vi "EnqueueError.vi"(8 "ErrorArray":errorcluster[](array[cluster])) -> (0 "ErrorArray":errorcluster[](array[cluster]))   [LabVIEW 2014, in "Bus_class.lvlib" / "Bus.lvclass"]
uses:
  Bus.lvclass
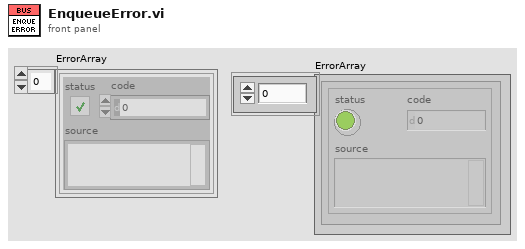
[diagram p1: front panel]
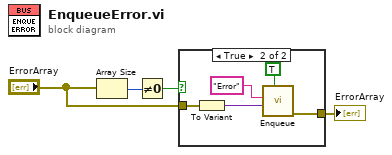
[diagram p0: block diagram]
diagram:
  n1 = Array Size(array="ErrorArray") -> (size(s)=w4:i32)
  n2 = Not Equal To 0?(x=w4) -> (x != 0?=w3:bool)
  n3 = case shown="True" w3 {
    tunnel: "ErrorArray" -> [_ w8]
    tunnel: [_ w5] -> w1
    frame False {
    }
    frame True {
      n4 = To Variant(anything=w8) -> (Variant=w9:variant)
      n5 = call "Enqueue.vi"("Priority (f)"=TRUE, "Data"=w9, "Msg"="Error") -> ("ErrorArray"=w5:errorcluster[])  [unwired: 8 in]
    }
  }
  "ErrorArray" <- w1
